vi "CommFlush(SubVI).vi"(8 "error in (no error)":errorcluster) -> (0 "error out":errorcluster)   [LabVIEW 2017, in "MainFrameLib.lvlib"]
uses:
  MainFrameLib.lvlib
  TypeDefs/FGV_Enum.ctl
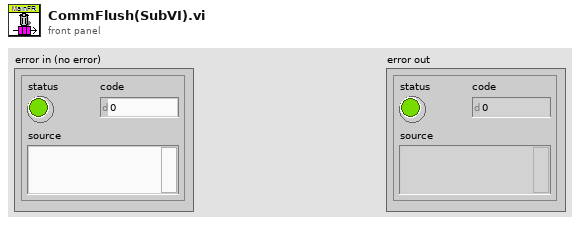
[diagram p1: front panel]
types:
  T1 = typedef "MainFrameLib.lvlib/FGV_Enum.ctl" = enum16{"Close", "GetRefs", "Initialize"}
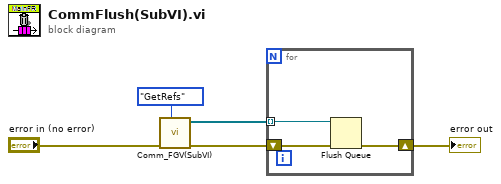
[diagram p0: block diagram]
diagram:
  n1 = call "Comm_FGV(SubVI).vi"("Enum"=FGV_Enum."GetRefs", "error in (no error)"="error in (no error)") -> ("error out"=w4:errorcluster, "Array"=w1:refnum<queue>[])  [unwired: 8 in]
  n2 = for {
    shift-right: [w7] -> w2
    shift-left: w4 -> [w8]
    tunnel: w1 -> [w6] mode=indexing
    n3 = Flush Queue(queue=w6, error in (no error)=w8) -> (error out=w7:errorcluster)  [unwired: 2 out]
  }
  "error out" <- w2
